vi "Query Status.vi"(0 "VISA resource name":refnum<visa-resource-name>, 11 "error in (no error)":errorcluster) -> (3 "Number of Pixels":u16, 4 "VISA resource name out":refnum<visa-resource-name>, 6 "Integration Time":u32, 8 "Packets in Spectra":u8, 10 "Packet Count":u8, 13 "Lamp Status":bool, 14 "USB Speed":u16(ring)=128 items=["Full Speed (12 Mbps)"=0, "High Speed (480 Mbps)"=128], 15 "error out":errorcluster)   [LabVIEW 2026, in "Ocean Optics 2000 4000.lvlib"]
doc: "Returns the intrument status information. Information included are number of pixels, intergration time, packets in spectra, packet count, USB speed and Lamp status.\n\n<B>Note:</b>\nNot supported by USB2000 and HR2000"
uses:
  Ocean Optics 2000 4000.lvlib
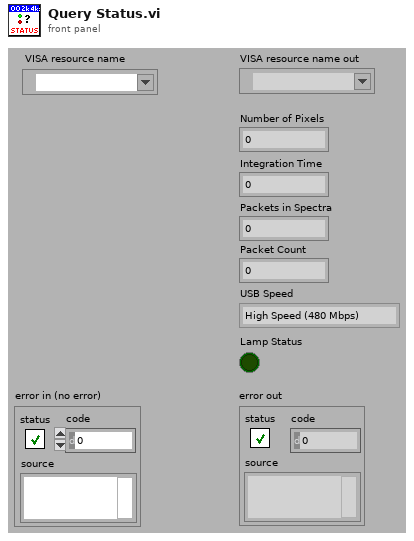
[diagram p1: front panel]
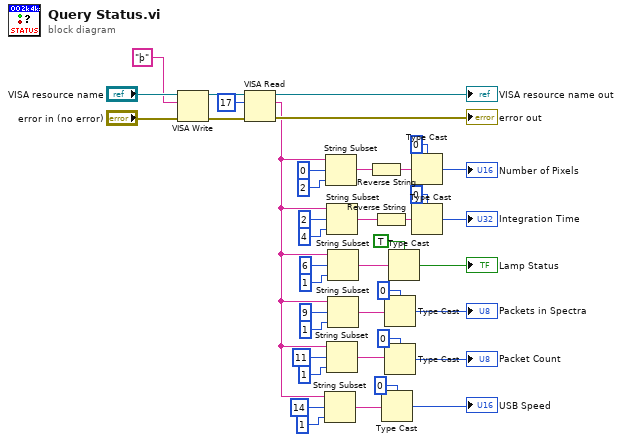
[diagram p0: block diagram]
diagram:
  n1 = VISA Write(VISA resource name="VISA resource name", write buffer="þ", error in (no error)="error in (no error)") -> (VISA resource name out=w37:refnum<visa-resource-name>, error out=w38:errorcluster)  [unwired: 1 out]
  n2 = VISA Read(VISA resource name=w37, byte count=u32 17, error in (no error)=w38) -> (VISA resource name out=→"VISA resource name out":refnum<visa-resource-name>, read buffer=w4:string, error out=→"error out":errorcluster)  [unwired: 1 out]
  n3 = String Subset(string=w4, offset (0)=14, length (rest)=1 ("length (rest)")) -> (substring=w2:string)
  n4 = String Subset(string=w4, offset (0)=0, length (rest)=2 ("length (rest)")) -> (substring=w30:string)
  n5 = String Subset(string=w4, offset (0)=2, length (rest)=4 ("length (rest)")) -> (substring=w25:string)
  n6 = String Subset(string=w4, offset (0)=11, length (rest)=1 ("length (rest)")) -> (substring=w8:string)
  n7 = String Subset(string=w4, offset (0)=6, length (rest)=1 ("length (rest)")) -> (substring=w19:string)
  n8 = String Subset(string=w4, offset (0)=9, length (rest)=1 ("length (rest)")) -> (substring=w14:string)
  n9 = Reverse String(1:w30) -> (0:w31:string)
  n10 = Reverse String(1:w25) -> (0:w22:string)
  n11 = Type Cast(type=u8 0, x=w2) -> (*(type *) &x=→"USB Speed":u8)
  n12 = Type Cast(type=u8 0, x=w14) -> (*(type *) &x=→"Packets in Spectra":u8)
  n13 = Type Cast(type=u8 0, x=w8) -> (*(type *) &x=→"Packet Count":u8)
  n14 = Type Cast(type=TRUE, x=w19) -> (*(type *) &x=→"Lamp Status":bool)
  n15 = Type Cast(type=u16 0, x=w31) -> (*(type *) &x=→"Number of Pixels":u16)
  n16 = Type Cast(type=u32 0, x=w22) -> (*(type *) &x=→"Integration Time":u32)
